vi "generate_artificial_neuron_config.vi"(3 "Analog Out Channels":cluster{"0":bool, "1":bool}={"0"=TRUE, "1"=FALSE}, 4 "Generate config":T1={"maximum value"=5.0, "minimum value"=-5.0, "phase"=180.0, "amplitude"=1.0, "frequency"=10.0, "Wave Type"=0, "offset"=0.0} {"offset" format="%0.2p"; "Wave Type" items=["Sine", "Square", "Triangle", "Sawtooth", "DC Signal"]; "frequency" format="%0.2p"; "amplitude" format="%0.2p"}, 5 "new task name":string) -> (0 "error out":errorcluster, 1 "signal Generated":waveform(dbl)(graph), 2 "task out":refnum<k21>)   [LabVIEW 2017]
uses:
  <vilib>/DAQmx/write.llb/DAQmx Write (Analog Wfm 1Chan NSamp).vi
  <vilib>/DAQmx/create/channels.llb/DAQmx Create Channel (AO-Voltage-Basic).vi
  <vilib>/DAQmx/configure/timing.llb/DAQmx Timing (Use Waveform).vi
  <vilib>/DAQmx/miscellaneous.llb/DAQmx Fill In Error Info.vi
  <instrlib>/NI USB-6356/NI USB-6356.lvlib
  <vilib>/ptbypt/NI_PtbyPt.lvlib
panel:
  out "number":u32
  out "sf (Hz)":dbl
  out "dt (s)":dbl
  in  "error in":errorcluster
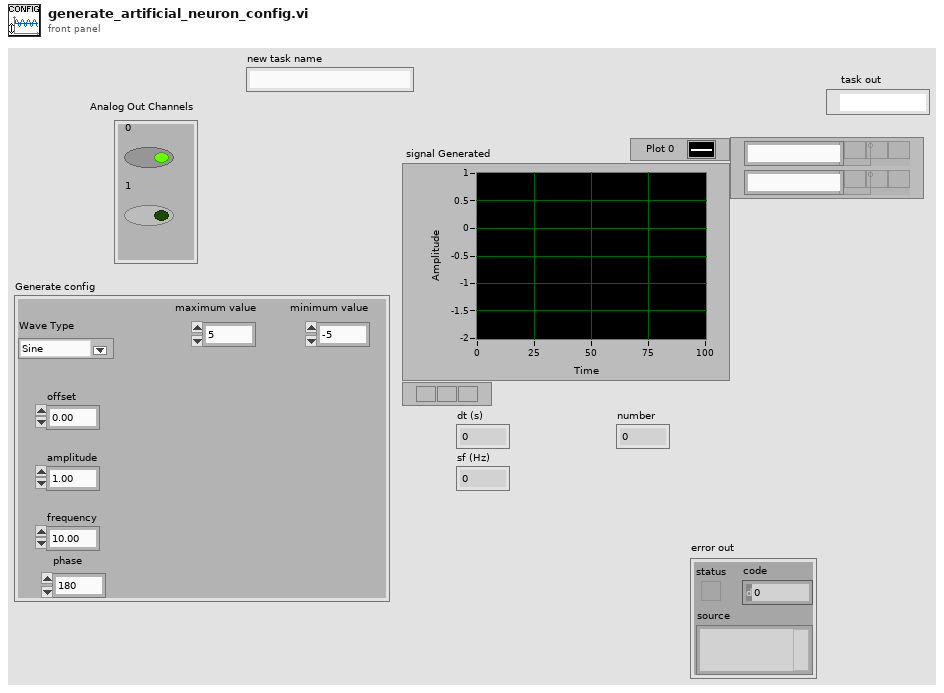
[diagram p1: front panel]
types:
  T1 = cluster{"maximum value":dbl, "minimum value":dbl, "phase":dbl, "amplitude":dbl, "frequency":dbl, "Wave Type":u16, "offset":dbl}
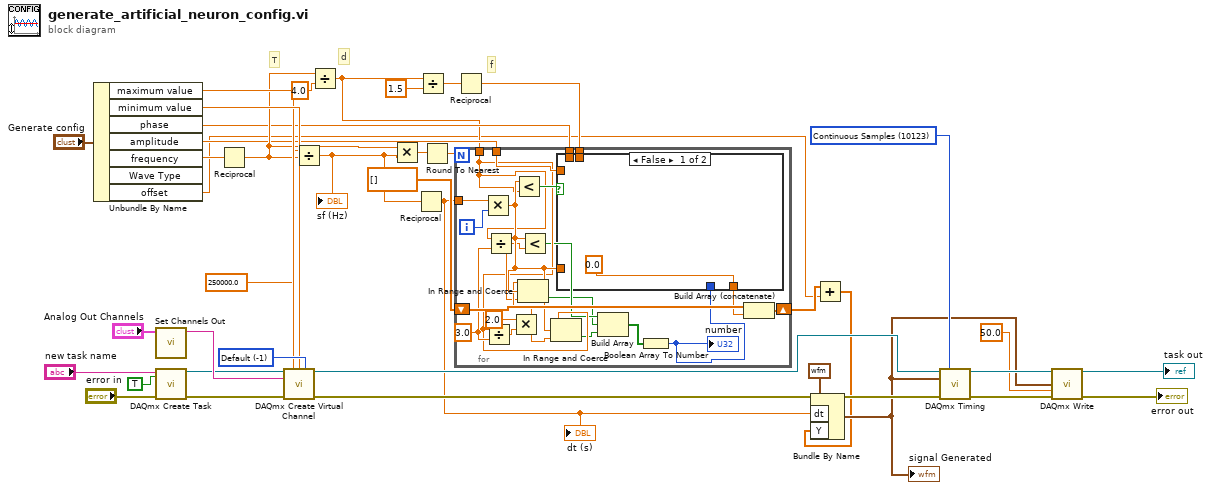
[diagram p0: block diagram]
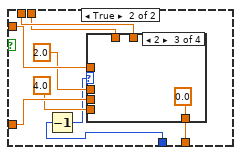
[diagram p2: hidden frame]
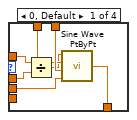
[diagram p3: hidden frame]
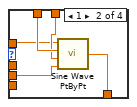
[diagram p4: hidden frame]
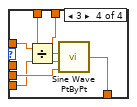
[diagram p5: hidden frame]
diagram:
  w34 = 10123 items=["Finite Samples"=10178, "Continuous Samples"=10123, "Hardware Timed Single Point"=12522] ("sample mode")
  w39 = -1 items=["Default"=-1, "RSE"=10083, "Differential"=10106, "Pseudodifferential"=12529] ("output terminal configuration")
  # "f"
  # "T"
  # "d"
  n1 = Unbundle By Name("Generate config") -> ("maximum value"=w23:dbl, "minimum value"=w24:dbl, "phase"=w9:dbl, "amplitude"=w8:dbl, "frequency"=w19:dbl, "offset"=w2:dbl)  [unwired: 1 out]
  n2 = call <instrlib>:"Set Channels Out.vi"("Analog Out Channels"="Analog Out Channels") -> ("String"=w38:string)  [unwired: 10 in]
  n3 = call <vilib>:"DAQmx Create Task.vi"("new task name"="new task name", "auto cleanup"=TRUE, "error in"="error in") -> ("task out"=w28:refnum<k21>, "error out"=w27:errorcluster)  [unwired: 11 in]
  n4 = Reciprocal(x=w19) -> (1/x=w10:dbl)
  n5 = call-poly <vilib>:"DAQmx Create Virtual Channel.vi"("task in"=w28, "maximum value"=w23, "minimum value"=w24, "output terminal configuration"=w39, "physical channels"=w38, "error in"=w27) -> ("task out"=w37:refnum<k21>, "error out"=w21:errorcluster)  [unwired: 8 in]
  n6 = Divide(x=250000.0, y=w10) -> (x/y=w11:dbl)
  "sf (Hz)" <- w11
  n7 = Divide(x=w10, y=4.0) -> (x/y=w6:dbl)
  n8 = Multiply(x=w10, y=w11) -> (x*y=w12:dbl)
  n9 = Reciprocal(x=w11) -> (1/x=w14:dbl)
  "dt (s)" <- w14
  n10 = Divide(x=w6, y=1.5) -> (x/y=w5:dbl)
  n11 = Round To Nearest(number=w12) -> (nearest integer value=w18:dbl)
  n12 = Reciprocal(x=w5) -> (1/x=w7:dbl)
  n13 = for {
    N: w18 -> [_]
    tunnel: w14 -> [w60]
    shift-right: [w57] -> w3
    shift-left: dbl[] [] -> [w58]
    tunnel: w6 -> [w45]
    tunnel: w9 -> [w55]
    tunnel: w7 -> [w54]
    tunnel: w8 -> [w53]
    i -> [w59]
    w49 = 3.0 ("y")
    n14 = Multiply(x=w60, y=w59) -> (x*y=w48:dbl)
    n15 = Divide(x=w45, y=w49) -> (x/y=w51:dbl)
    n16 = Divide(x=w45, y=w49) -> (x/y=w46:dbl)
    n17 = Multiply(x=2.0, y=w51) -> (x*y=w47:dbl)
    n18 = Less?(x=w48, y=w45) -> (x < y?=w56:bool)
    n19 = In Range and Coerce(upper limit=w47, x=w48, lower limit=w46) -> (In Range?=w43:bool)  [unwired: 1 out]
    n20 = Less?(x=w48, y=w46) -> (x < y?=w44:bool)
    n21 = In Range and Coerce(upper limit=w45, x=w48, lower limit=w47) -> (In Range?=w42:bool)  [unwired: 1 out]
    n22 = Build Array(w44, w43, w42) -> (w41:bool[])
    n23 = Boolean Array To Number(Boolean array=w41) -> (number=w40:u32)
    "number" <- w40
    n24 = case shown="False" w56 {
      tunnel: w48 -> [_ w70]
      tunnel: w55 -> [_ w69]
      tunnel: w54 -> [_ w68]
      tunnel: w53 -> [_ w66]
      tunnel: [0.0 ("sine wave") w67] -> w52
      tunnel: w40 -> [_ w63]
      frame False {
      }
      frame True {
        n25 = Decrement(x=w63) -> (x-1=w62:u32)
        n26 = case shown="2" w62 {
          tunnel: w70 -> [w77 w80 _ w89]
          tunnel: w69 -> [w76 w81 _ w87]
          tunnel: w68 -> [w75 w82 _ w88]
          tunnel: [w74 w79 0.0 ("sine wave") w90] -> w67
          tunnel: w66 -> [w73 w78 _ w86]
          tunnel: 2.0 ("y") -> [w72 _ _ _]
          tunnel: 4.0 ("y") -> [_ _ _ w85]
          frame 0, Default {
            n27 = Divide(x=w73, y=w72) -> (x/y=w71:dbl)
            n28 = call <vilib>:"Sine Wave PtByPt.vi"("time"=w77, "phase"=w76, "frequency"=w75, "amplitude"=w71) -> ("sine wave"=w74:dbl)
          }
          frame 1 {
            n29 = call <vilib>:"Sine Wave PtByPt.vi"("time"=w80, "phase"=w81, "frequency"=w82, "amplitude"=w78) -> ("sine wave"=w79:dbl)
          }
          frame 2 {
          }
          frame 3 {
            n30 = Divide(x=w86, y=w85) -> (x/y=w84:dbl)
            n31 = call <vilib>:"Sine Wave PtByPt.vi"("time"=w89, "phase"=w87, "frequency"=w88, "amplitude"=w84) -> ("sine wave"=w90:dbl)
          }
        }
      }
    }
    n32 = Build Array (concatenate)(w58, w52) -> (w57:dbl[])
  }
  n33 = Add(x=w3, y=w2) -> (x+y=w1:dbl[])
  n34 = Bundle By Name(cluster=waveform(dbl) {"t0"=timestamp(0 s since 1904-01-01), "dt"=1.0, "Y"=[]} ("waveform"), "dt"=w14, "Y"=w1) -> (w20:waveform(dbl))
  "signal Generated" <- w20
  n35 = call-poly <vilib>:"DAQmx Timing.vi"("task/channels in"=w37, "sample mode"=w34, "waveform"=w20, "error in"=w21) -> ("task out"=w35:refnum<k21>, "error out"=w36:errorcluster)  [unwired: 10 in]
  n36 = call-poly <vilib>:"DAQmx Write.vi"("task/channels in"=w35, "data"=w20, "timeout"=50.0, "error in"=w36) -> ("task out"=→"task out":refnum<k21>, "error out"=→"error out":errorcluster)  [unwired: 9 in, 1 out]
